vi "save-autofocus-global.vi"() -> ()   [LabVIEW 2014]
panel:
  in  "Load File":path
  out "Filename":string
  out "Save current?":bool
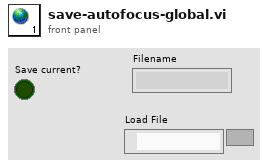
[diagram p1: front panel]
diagram:
